vi "按钮旋转子vi100-200.vi"(9 "Ctl引用句柄":refnum<vi>) -> ()   [LabVIEW 2018]
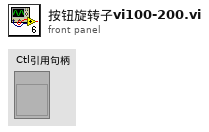
[diagram p1: front panel]
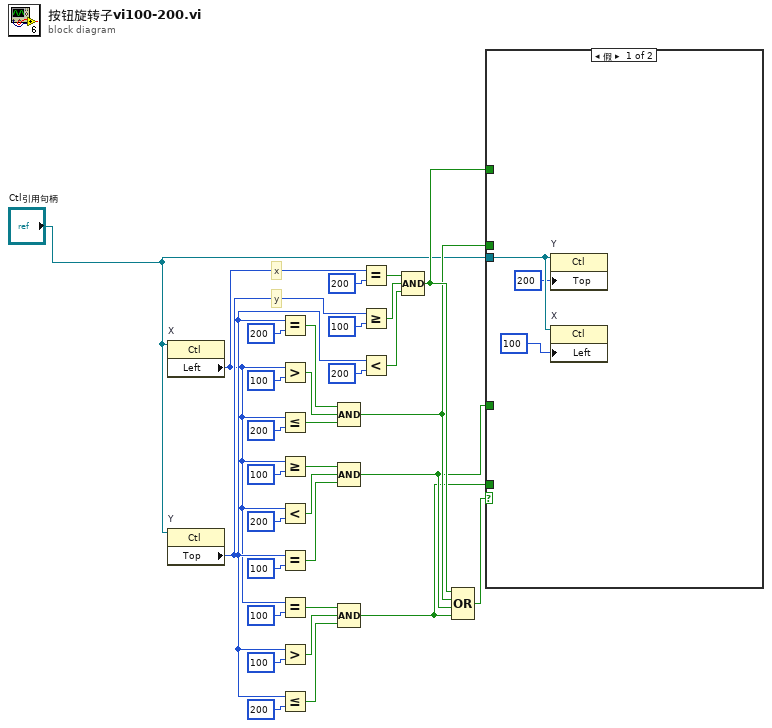
[diagram p0: block diagram]
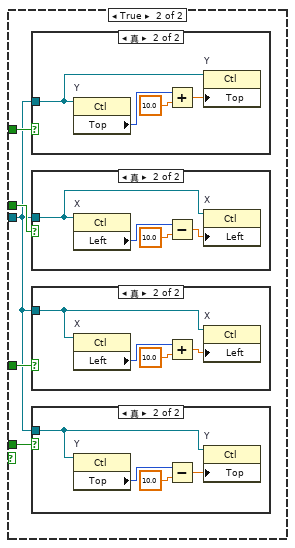
[diagram p2: hidden frame]
diagram:
  # "y"
  # "x"
  n1 = property on="X" class="Ctl"(reference="Ctl引用句柄") -> ("Left"=w5:i32)  [unwired: 1 in, 2 out]
  n2 = property on="Y" class="Ctl"(reference="Ctl引用句柄") -> ("Top"=w6:i32)  [unwired: 1 in, 2 out]
  n3 = Equal?(x=w6, y=200) -> (x = y?=w17:bool)
  n4 = Greater?(x=w5, y=100) -> (0:w16:bool)
  n5 = Less Or Equal?(x=w5, y=200) -> (x <= y?=w15:bool)
  n6 = Greater Or Equal?(x=w5, y=100) -> (x >= y?=w29:bool)
  n7 = Less?(x=w5, y=200) -> (x < y?=w28:bool)
  n8 = Equal?(x=w6, y=100) -> (x = y?=w27:bool)
  n9 = Equal?(x=w5, y=100) -> (x = y?=w11:bool)
  n10 = Greater?(x=w6, y=100) -> (0:w10:bool)
  n11 = Less Or Equal?(x=w6, y=200) -> (x <= y?=w9:bool)
  n12 = Compound Arithmetic op=AND ("复合运算")(w17, w16, w15) -> (w4:bool)
  n13 = Compound Arithmetic op=AND ("复合运算")(w29, w28, w27) -> (w3:bool)
  n14 = Compound Arithmetic op=AND ("复合运算")(w11, w10, w9) -> (w2:bool)
  n15 = Equal?(x=w5, y=200) -> (x = y?=w23:bool)
  n16 = Greater Or Equal?(x=w6, y=100) -> (x >= y?=w22:bool)
  n17 = Less?(x=w6, y=200) -> (x < y?=w21:bool)
  n18 = Compound Arithmetic op=AND ("复合运算")(w23, w22, w21) -> (w7:bool)
  n19 = Compound Arithmetic op=OR ("复合运算")(w7, w4, w3, w2) -> (w8:bool)
  n20 = case shown="假" w8 {
    tunnel: "Ctl引用句柄" -> [w35 w36]
    tunnel: w7 -> [_ w40]
    tunnel: w3 -> [_ w39]
    tunnel: w4 -> [_ w38]
    tunnel: w2 -> [_ w37]
    frame False {
      n21 = property on="Y" class="Ctl"(reference=w35, "Top"=200 ("位置:置顶")) -> ()  [unwired: 1 in, 2 out]
      n22 = property on="X" class="Ctl"(reference=w35, "Left"=100) -> ()  [unwired: 1 in, 2 out]
    }
    frame True {
      n23 = case shown="真" w40 {
        tunnel: w36 -> [_ w53]
        frame False {
        }
        frame True {
          n24 = property on="Y" class="Ctl"(reference=w53) -> ("Top"=w54:i32)  [unwired: 1 in, 2 out]
          n25 = Add(x=w54, y=10.0) -> (x+y=w56:dbl)
          n26 = property on="Y" class="Ctl"(reference=w53, "Top"=w56) -> ()  [unwired: 1 in, 2 out]
        }
      }
      n27 = case shown="真" w38 {
        tunnel: w36 -> [_ w49]
        frame False {
        }
        frame True {
          n28 = property on="X" class="Ctl"(reference=w49) -> ("Left"=w51:i32)  [unwired: 1 in, 2 out]
          n29 = Subtract(x=w51, y=10.0) -> (x-y=w50:dbl)
          n30 = property on="X" class="Ctl"(reference=w49, "Left"=w50) -> ()  [unwired: 1 in, 2 out]
        }
      }
      n31 = case shown="真" w39 {
        tunnel: w36 -> [_ w45]
        frame False {
        }
        frame True {
          n32 = property on="X" class="Ctl"(reference=w45) -> ("Left"=w47:i32)  [unwired: 1 in, 2 out]
          n33 = Add(x=w47, y=10.0) -> (x+y=w46:dbl)
          n34 = property on="X" class="Ctl"(reference=w45, "Left"=w46) -> ()  [unwired: 1 in, 2 out]
        }
      }
      n35 = case shown="真" w37 {
        tunnel: w36 -> [_ w41]
        frame False {
        }
        frame True {
          n36 = property on="Y" class="Ctl"(reference=w41) -> ("Top"=w42:i32)  [unwired: 1 in, 2 out]
          n37 = Subtract(x=w42, y=10.0) -> (x-y=w44:dbl)
          n38 = property on="Y" class="Ctl"(reference=w41, "Top"=w44) -> ()  [unwired: 1 in, 2 out]
        }
      }
    }
  }
